vi "Check if test passed or failed.vi"(8 "error in (no error)":errorcluster, 11 "Message":string) -> (0 "error out":errorcluster, 2 "Passed?":bool, 3 "Measurement":string)   [LabVIEW 2013]
uses:
  <vilib>/event_ctls.llb/eventvkey.ctl
panel:
  in  "Failed":bool
  in  "Passed":bool
  # "Operator Message"
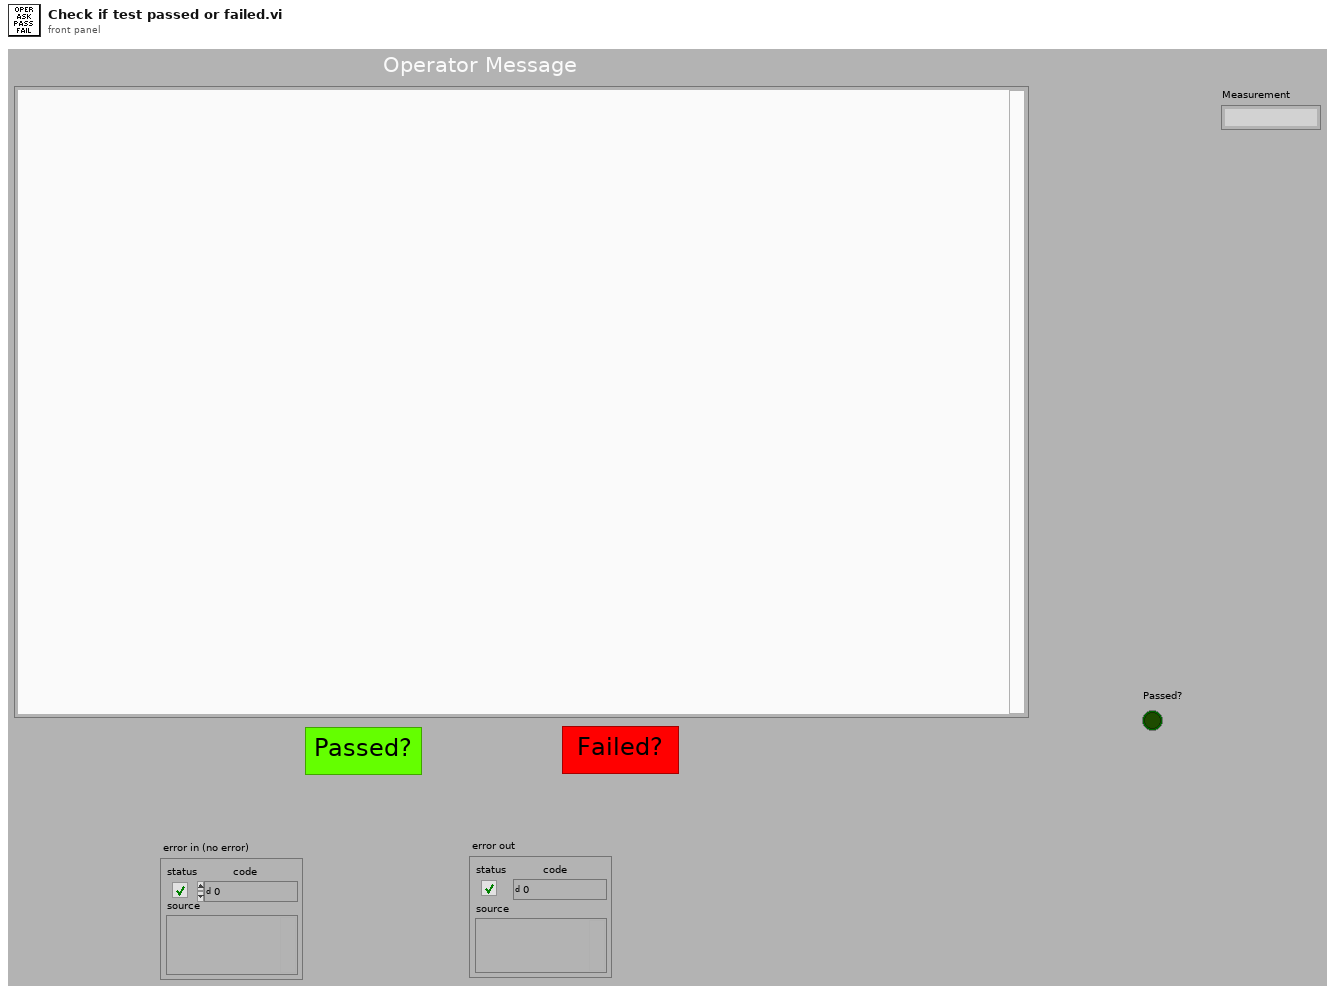
[diagram p1: front panel]
types:
  T1 = typedef "eventvkey.ctl" = enum16{"ASCII", "Enter", "Return", "Shift", "Ctrl", "Alt", "Cmd", "Opt", "Caps", "NumLock", "Clear", "Break", "Up", "Down", "Left", "Right", "Insert", "Delete", "Home", "End", "PageUp", "PageDown", "Escape", "Help", "Pause", "ScrollLock", "F1", "F2", "F3", "F4", "F5", "F6", "F7", "F8", "F9", "F10", "F11", "F12", "F13", "F14", "F15", "F16", "F17", "F18", "F19", "F20", "F21", "F22", "F23", "F24", "Play", "VolumeUp", "VolumeDown", "Mute", "Two Byte Char"}
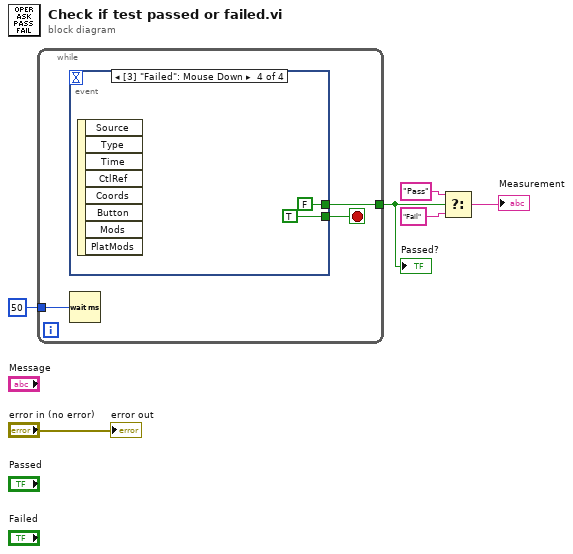
[diagram p0: block diagram]
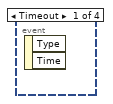
[diagram p2: hidden frame]
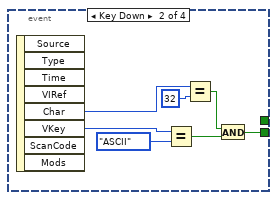
[diagram p3: hidden frame]
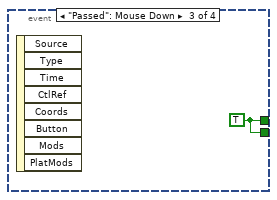
[diagram p4: hidden frame]
diagram:
  n1 = while {
    tunnel: u32 50 ("milliseconds to wait") -> [w9]
    tunnel: [w7] -> w4
    stop <- w8 stop-if-true
    n2 = event shown="[3] \"Failed\": Mouse Down" {
      selector: _ -> [_ _ _ _]
      dyn-events: _ -> [_ _ _ _]
      timeout: _ -> [_ _ _ _]
      tunnel: [_ w10 w17 TRUE] -> w8
      tunnel: [_ _ w17 FALSE] -> w7
      event Timeout {
        n3 = event-data() -> ()  [unwired: 1 in, 2 out]
      }
      event Key Down {
        n4 = event-data() -> ("Char"=w16:i16, "VKey"=w14:T1)  [unwired: 1 in, 6 out]
        n5 = Equal?(x=w14, y=eventvkey."ASCII" ("VKey")) -> (x = y?=w11:bool)
        n6 = Equal?(x=w16, y=i16 32) -> (x = y?=w12:bool)
        n7 = And(x=w12, y=w11) -> (x .and. y?=w10:bool)
      }
      event "Passed": Mouse Down {
        w17 = TRUE
        n8 = event-data() -> ()  [unwired: 1 in, 8 out]
      }
      event "Failed": Mouse Down {
        n9 = event-data() -> ()  [unwired: 1 in, 8 out]
      }
    }
    n10 = Wait (ms)(milliseconds to wait=w9) -> ()  [unwired: 1 out]
  }
  "Passed?" <- w4
  n11 = Select(t="Pass", s=w4, f="Fail") -> (s? t:f=→"Measurement":string)
  "error out" <- "error in (no error)"
